vi "mark_253.vi"(9 "mark value":i32=1, 10 "Memory in 2":T1, 11 "Memory in":T1) -> (2 "action":T2, 3 "Memory out":T1)   [LabVIEW 2015, in "PolyVIEW.lvclass"]
uses:
  PolyVIEW.lvclass
  ant_base/action_cluster.ctl
  ant_base/actionType_enum.ctl
  Memory.ctl
  ant_base/ant_base.lvclass
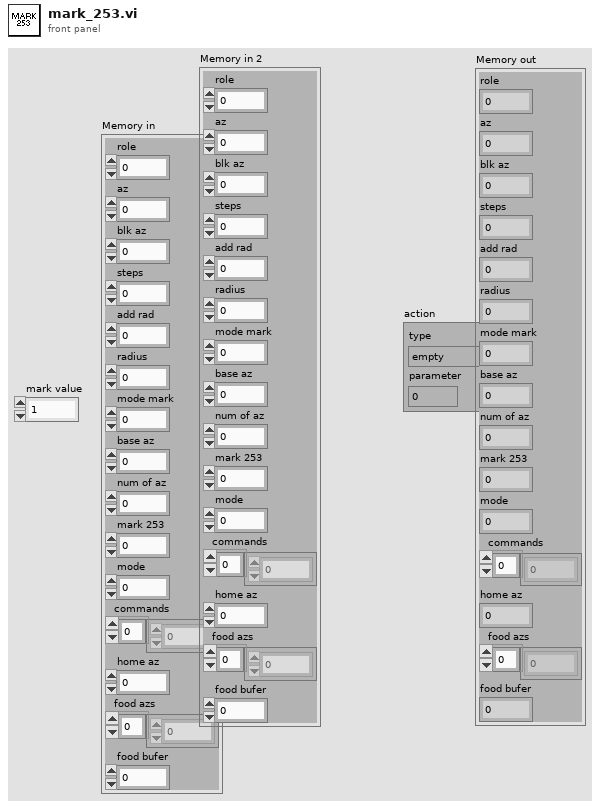
[diagram p1: front panel]
types:
  T1 = typedef "PolyVIEW.lvclass/Memory.ctl" = cluster{"role":i32, "az":i32, "blk az":i32, "steps":u32, "add rad":i32, "radius":dbl, "mode mark":u32, "base az":dbl, "num of az":u32, "mark 253":u32, "mode":u32, "commands":i32[], "home az":dbl, "food azs":dbl[], "food bufer":dbl}
  T2 = typedef "ant_base.lvclass/action_cluster.ctl" = cluster{"type":T3, "parameter":dbl}
  T3 = typedef "ant_base.lvclass/actionType_enum.ctl" = enum8{"empty", "move", "take", "put", "mark"}
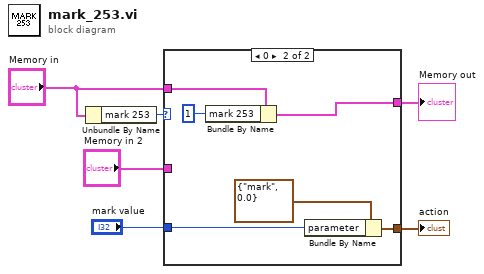
[diagram p0: block diagram]
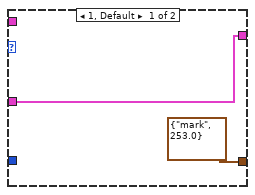
[diagram p2: hidden frame]
diagram:
  n1 = Unbundle By Name("Memory in") -> ("mark 253"=w4:u32)
  n2 = case shown="0" w4 {
    tunnel: [T2 {"type"=enum."mark", "parameter"=253.0} ("action") w14] -> w6
    tunnel: "Memory in" -> [_ w11]
    tunnel: [w7 w9] -> w1
    tunnel: "Memory in 2" -> [w7 _]
    tunnel: "mark value" -> [_ w12]
    frame 1, Default {
    }
    frame 0 {
      n3 = Bundle By Name(cluster=w11, "mark 253"=u8 1 ("new element/subarray")) -> (w9:T1)
      n4 = Bundle By Name(cluster=T2 {"type"=enum."mark", "parameter"=0.0} ("action"), "parameter"=w12) -> (w14:T2)
    }
  }
  "action" <- w6
  "Memory out" <- w1
